vi "100ms loop.vi"() -> ()   [LabVIEW 2012]
uses:
  <vilib>/Rock Robotics/WPI/Relay/WPI_RelayValue.ctl
panel:
  in  "LED on":bool=TRUE
  in  "Compressor Off":bool
  out "Pressure Met":bool=TRUE
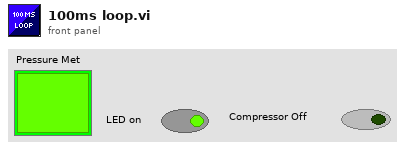
[diagram p1: front panel]
types:
  T1 = typedef "WPI_RelayValue.ctl" = enum16{"Off", "On", "Forward", "Reverse"}
  T2 = typedef "WPI_DigitalInputDevRef.ctl" = cluster{"DevStatus":errorcluster, "DIO Channel":T3, "Digital Module":T4}
  T3 = typedef "FPGA_DIOChannel.ctl" = enum8{"DIO 1", "DIO 2", "DIO 3", "DIO 4", "DIO 5", "DIO 6", "DIO 7", "DIO 8", "DIO 9", "DIO 10", "DIO 11", "DIO 12", "DIO 13", "DIO 14", "Invalid"}
  T4 = typedef "FPGA_TypedefDigitalModule.ctl" = enum16{"Digital Module 1", "Digital Module 2"}
  T5 = typedef "WPI_RelayDevRef.ctl" = cluster{"DevStatus":errorcluster, "Relay Channel":T6, "Digital Module":T4, "Relay Direction":T7}
  T6 = typedef "FPGA_DIORelayChannel.ctl" = enum8{"Relay 1", "Relay 2", "Relay 3", "Relay 4", "Relay 5", "Relay 6", "Relay 7", "Relay 8", "Invalid"}
  T7 = typedef "WPI_RelayDirection.ctl" = enum16{"Both directions", "Forward only", "Reverse only"}
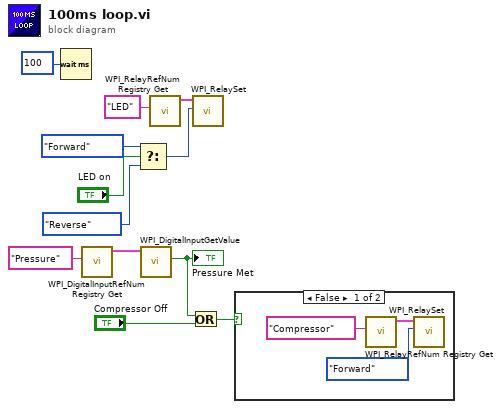
[diagram p0: block diagram]
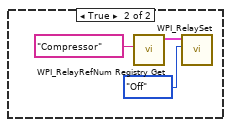
[diagram p2: hidden frame]
diagram:
  n1 = Wait (ms)(milliseconds to wait=u32 100) -> ()  [unwired: 1 out]
  n2 = call <vilib>:"WPI_DigitalInputRefNum Registry Get.vi"("refnum name"="Pressure") -> ("DigitalInputDevRef"=w11:T2)  [unwired: 9 in, 1 out]
  n3 = Select(t=WPI_RelayValue."Forward" ("RelayValue"), s="LED on", f=WPI_RelayValue."Reverse") -> (s? t:f=w3:T1)
  n4 = call <vilib>:"WPI_DigitalInputGetValue.vi"("DigitalInputDevRef"=w11) -> ("Value"=w9:bool)  [unwired: 8 in, 2 out]
  "Pressure Met" <- w9
  n5 = call <vilib>:"WPI_RelayRefNum Registry Get.vi"("refnum name"="LED") -> ("RelayDevRef"=w6:T5)  [unwired: 9 in, 1 out]
  n6 = Or(x=w9, y="Compressor Off") -> (x .or. y?=w8:bool)
  n7 = call <vilib>:"WPI_RelaySet.vi"("RelayValue"=w3, "RelayDevRef"=w6) -> ()  [unwired: 8 in, 2 out]
  n8 = case shown="False" w8 {
    frame False {
      n9 = call <vilib>:"WPI_RelayRefNum Registry Get.vi"("refnum name"="Compressor") -> ("RelayDevRef"=w15:T5)  [unwired: 9 in, 1 out]
      n10 = call <vilib>:"WPI_RelaySet.vi"("RelayValue"=WPI_RelayValue."Forward", "RelayDevRef"=w15) -> ()  [unwired: 8 in, 2 out]
    }
    frame True {
      n11 = call <vilib>:"WPI_RelayRefNum Registry Get.vi"("refnum name"="Compressor") -> ("RelayDevRef"=w18:T5)  [unwired: 9 in, 1 out]
      n12 = call <vilib>:"WPI_RelaySet.vi"("RelayValue"=WPI_RelayValue."Off", "RelayDevRef"=w18) -> ()  [unwired: 8 in, 2 out]
    }
  }
